vi "iWorx Snapshot.vi"(8 "Error In":errorcluster, 11 "WaveformChart in":refnum<vi>) -> (0 "Error Out":errorcluster)   [LabVIEW 2012]
doc: "This VI is designed to take a screenshot of a waveform chart (specified by reference), and prompt to user to save it on disc."
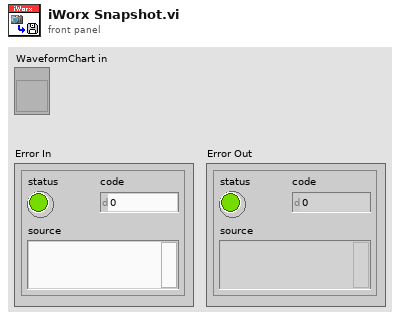
[diagram p1: front panel]
types:
  T1 = enum16{"open", "replace", "create", "open or create", "replace or create", "replace or create with confirmation"}
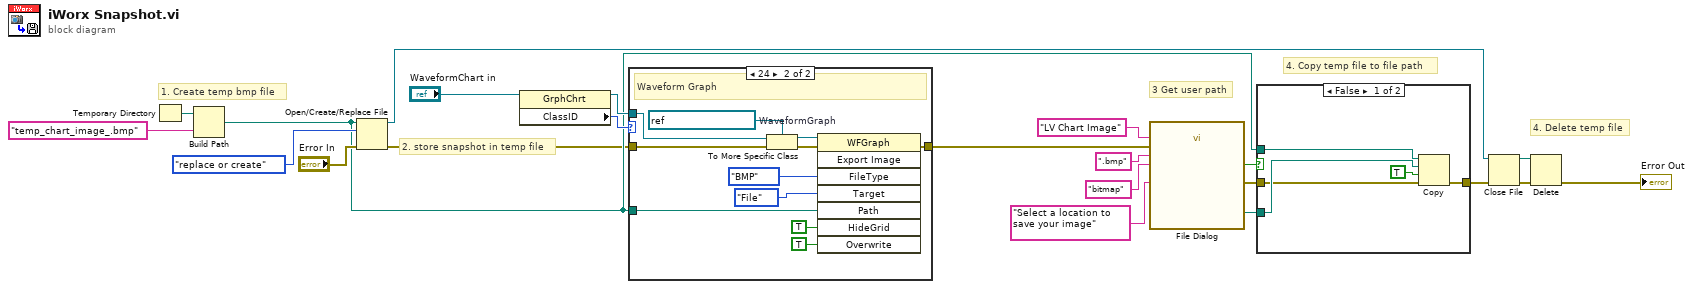
[diagram p0: block diagram]
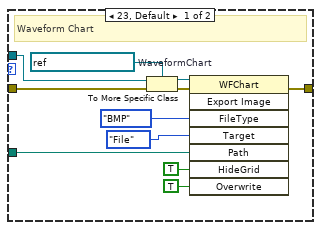
[diagram p2: hidden frame]
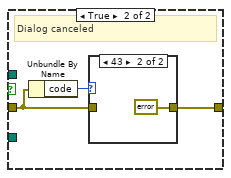
[diagram p3: hidden frame]
diagram:
  # "3 Get user path"
  # "4. Delete temp file"
  # "4. Copy temp file to file path"
  # "2. store snapshot in temp file"
  # "1. Create temp bmp file"
  n1 = Temporary Directory() -> (w10:path)
  n2 = Build Path(base path=w10, name or relative path="temp_chart_image_.bmp") -> (appended path=w3:path)
  n3 = Open/Create/Replace File(file path (use dialog)=w3, error in="Error In", operation (0:open)=T1."replace or create") -> (refnum out=w14:refnum<file>, error out=w2:errorcluster)  [unwired: 3 in, 1 out]
  n4 = property class="GrphChrt"(reference="WaveformChart in") -> (reference out=w4:refnum<vi>, "ClassID"=w5:u32)  [unwired: 1 in, 1 out]
  n5 = case shown="24" w5 {
    tunnel: w4 -> [w33 w43]
    tunnel: w3 -> [w25 w35]
    tunnel: w2 -> [w24 w42]
    tunnel: [w23 w34] -> w1
    frame 23, Default {
      w32 = refnum<vi> refnum  # WaveformChart
      # "Waveform Chart"
      n6 = To More Specific Class(target class=w32, reference=w33, error in=w24) -> (specific class reference=w27:refnum<vi>, error out=w26:errorcluster)
      n7 = invoke on="Invoke Node" class="WFChart" method="Export Image"(reference=w27, error in=w26, "FileType"=enum32{"BMP", "EPS", "EMF", "PICT"}."BMP" ("File Type"), "Target"=enum32{"File", "Clipboard"}."File", "Path"=w25, "HideGrid"=TRUE ("Hide Grid"), "Overwrite"=TRUE ("Always Overwrite")) -> (error out=w23:errorcluster)  [unwired: 1 in, 7 out]
    }
    frame 24 {
      w44 = refnum<vi> refnum  # WaveformGraph
      # "Waveform Graph"
      n8 = To More Specific Class(target class=w44, reference=w43, error in=w42) -> (specific class reference=w40:refnum<vi>, error out=w41:errorcluster)
      n9 = invoke on="Invoke Node" class="WFGraph" method="Export Image"(reference=w40, error in=w41, "FileType"=enum32{"BMP", "EPS", "EMF", "PICT"}."BMP" ("File Type"), "Target"=enum32{"File", "Clipboard"}."File", "Path"=w35, "HideGrid"=TRUE ("Hide Grid"), "Overwrite"=TRUE ("Always Overwrite")) -> (error out=w34:errorcluster)  [unwired: 1 in, 7 out]
    }
  }
  n10 = call "File Dialog"("prompt"="Select a location to save your image", "default name"="LV Chart Image", "error in"=w1, "pattern (all files)"=".bmp", "pattern label"="bitmap") -> ("selected path"=w16:path, "cancelled"=w9:bool, "error out"=w15:errorcluster)  [unwired: 7 in, 1 out]
  n11 = case shown="False" w9 {
    tunnel: w3 -> [w49 _]
    tunnel: w16 -> [w48 _]
    tunnel: w15 -> [w47 w51]
    tunnel: [w46 w50] -> w13
    frame False {
      n12 = Copy(8:w47, 9:TRUE ("overwrite (F)"), 10:w48, 11:w49) -> (0:w46:errorcluster)  [unwired: 1 in, 2 out]
    }
    frame True {
      # "Dialog canceled"
      n13 = Unbundle By Name(w51) -> ("code"=w52:i32)
      n14 = case shown="43" w52 {
        tunnel: w51 -> [w53 _]
        tunnel: [w53 errorcluster {"status"=FALSE, "code"=0, "source"=""} ("error out")] -> w50
        frame 0, Default {
        }
        frame 43 {
        }
      }
    }
  }
  n15 = Close File(refnum=w14, error in=w13) -> (path=w12:path, error out=w11:errorcluster)
  n16 = Delete(path (use dialog)=w12, error in=w11) -> (error out=→"Error Out":errorcluster)  [unwired: 3 in, 2 out]
